vi "Load Config INI from File.vi"(7 "File Type":string(combo)=".gif", 8 "Error In":errorcluster, 10 "reference":refnum<vi>, 11 "Path In":path) -> (0 "Error Out":errorcluster, 3 "Path Out":path)   [LabVIEW 2015]
uses:
  <vilib>/Utility/config.llb/Read Key (String).vi
  <vilib>/Utility/config.llb/NI_LVConfig.lvlib
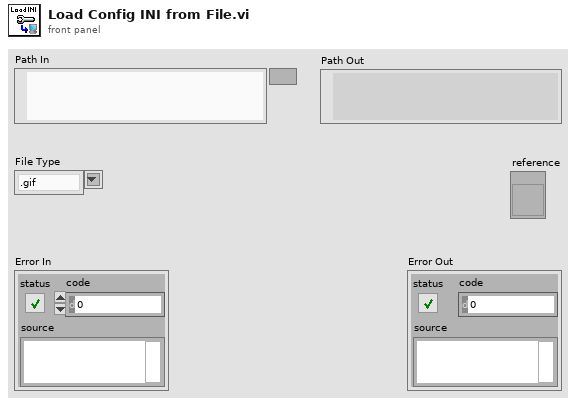
[diagram p1: front panel]
types:
  T1 = typedef "NI_LVConfig.lvlib/Config Data RefNum.ctl" = refnum<k1>
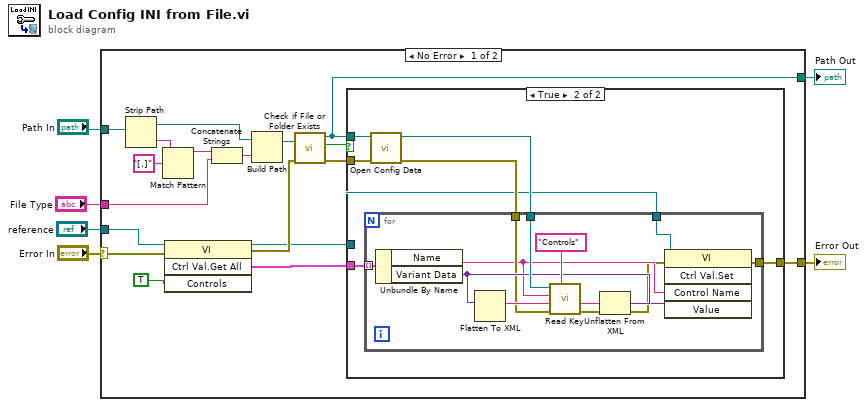
[diagram p0: block diagram]
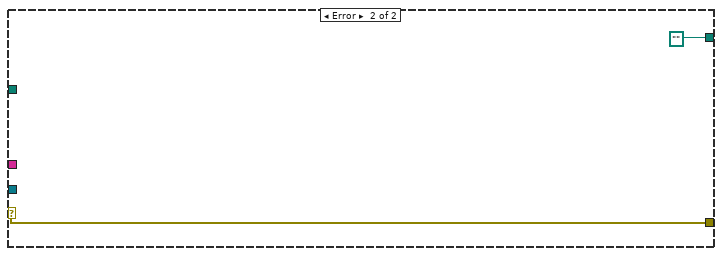
[diagram p3: hidden frame]
diagram:
  n1 = case shown="No Error" "Error In" {
    selector: "Error In" -> [w15 w47]
    tunnel: [w11 w47] -> w4
    tunnel: [w9 path ""] -> w3
    tunnel: "Path In" -> [w10 _]
    tunnel: "reference" -> [w8 _]
    tunnel: "File Type" -> [w7 _]
    frame No Error {
      n2 = Strip Path(path=w10) -> (stripped path=w19:path, name=w24:string)
      n3 = Match Pattern(string=w24, regular expression="[.]" ("search string")) -> (before substring=w22:string)  [unwired: 1 in, 3 out]
      n4 = invoke class="VI" method="Ctrl Val.Get All"(reference=w8, error in=w15, "Controls"=TRUE) -> (reference out=w12:refnum<vi>, error out=w14:errorcluster, "Get All Control Values Variant"=w13:cluster{"Name":string, "Variant Data":variant}[])  [unwired: 1 in, 1 out]
      n5 = Concatenate Strings(w22, w7) -> (w21:string)
      n6 = Build Path(base path=w19, name or relative path=w21) -> (appended path=w20:path)
      n7 = call <vilib>:"Check if File or Folder Exists.vi"("error in (no error)"=w14, "path"=w20) -> ("error out"=w17:errorcluster, "file or folder exists?"=w18:bool, "dup path"=w9:path)  [unwired: 7 in]
      n8 = case shown="True" w18 {
        tunnel: w9 -> [_ w32]
        tunnel: w17 -> [w25 w31]
        tunnel: w13 -> [_ w30]
        tunnel: w12 -> [_ w27]
        tunnel: [w25 w26] -> w11
        frame False {
        }
        frame True {
          n9 = call <vilib>:"Open Config Data.vi"("error in (no error)"=w31, "configuration file path"=w32) -> ("error out"=w28:errorcluster, "refnum"=w29:T1)  [unwired: 1 in, 7 out]
          n10 = for {
            tunnel: w30 -> [w44] mode=indexing
            tunnel: w29 -> [w43]
            tunnel: w28 -> [w39]
            tunnel: w27 -> [w37]
            tunnel: [w33] -> w26
            n11 = Unbundle By Name(w44) -> ("Name"=w36:string, "Variant Data"=w41:variant)
            n12 = Flatten To XML(anything=w41) -> (xml string=w42:string)
            n13 = call-poly <vilib>:"Read Key.vi"("section"="Controls", "error in (no error)"=w39, "default value"=w42, "key"=w36, "refnum"=w43) -> ("error out"=w38:errorcluster, "value"=w40:string)  [unwired: 3 in, 2 out]
            n14 = Unflatten From XML(xml string=w40, type=w41, error in (no error)=w38) -> (value=w35:variant, error out=w34:errorcluster)
            n15 = invoke class="VI" method="Ctrl Val.Set"(reference=w37, error in=w34, "Control Name"=w36, "Value"=w35) -> (error out=w33:errorcluster)  [unwired: 1 in, 4 out]
          }
        }
      }
    }
    frame Error {
      (unwired) ""
    }
  }
  "Error Out" <- w4
  "Path Out" <- w3
